vi "Save_Destinations.vi"(8 "error in (no error)":errorcluster, 11 "Installer in":refnum<class "Installer.lvclass">) -> (0 "error out":errorcluster, 3 "Installer out":refnum<class "Installer.lvclass">)   [LabVIEW 2020, in "Installer.lvclass"]
uses:
  <vilib>/AppBuilder/IB_Classes/Installer/Installer.lvclass
  <vilib>/AppBuilder/IB_Classes/Installer/Installer.lvclass/Installer.ctl
  <vilib>/AppBuilder/IB_Classes/Destination/IB_Destination.lvclass
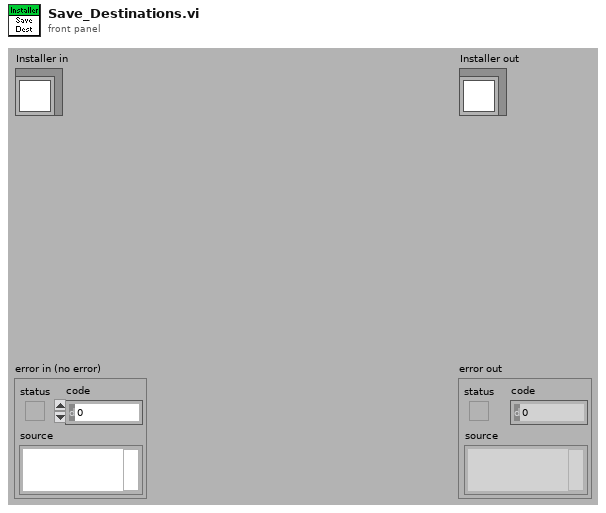
[diagram p1: front panel]
types:
  T1 = typedef "ItemRef.ctl" = u64
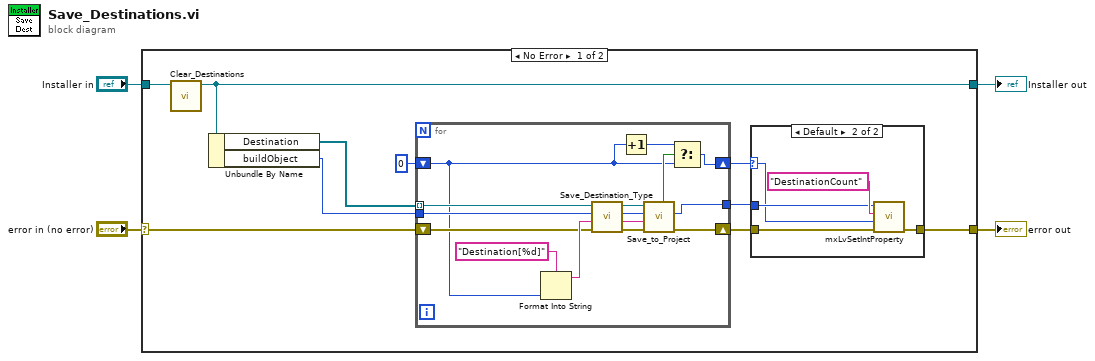
[diagram p0: block diagram]
diagram:
  n1 = case shown="No Error" "error in (no error)" {
    selector: "error in (no error)" -> [w7 w37]
    tunnel: [w6 w37] -> w3
    tunnel: [w12 w36] -> w1
    tunnel: "Installer in" -> [w13 w36]
    frame No Error {
      n2 = call <vilib>:"Clear_Destinations.vi"("Installer in"=w13) -> ("Installer out"=w12:refnum<class "Installer.lvclass">)  [unwired: 9 in, 1 out]
      n3 = Unbundle By Name(w12) -> ("Destination"=w14:refnum<class "IB_Destination.lvclass">[], "buildObject"=w11:T1)
      n4 = for {
        tunnel: w14 -> [w35] mode=indexing
        tunnel: w11 -> [w30]
        shift-right: [w27] -> w9
        shift-left: 0 -> [w21]
        shift-right: [w24] -> w8
        shift-left: w7 -> [w26]
        tunnel: [w23] -> w5
        n5 = Format Into String(format string="Destination[%d]", w21) -> (resulting string=w32:string)  [unwired: 2 in, 1 out]
        n6 = call-dynamic "Save_Destination_Type.vi"("error in (no error)"=w26, "index"=w32, "buildObject"=w30, "IB_Destination in"=w35) -> ("error out"=w25:errorcluster, "index out"=w31:string, "buildObject out"=w29:T1, "IB_Destination out"=w34:refnum<class "IB_Destination.lvclass">)  [unwired: 4 in]
        n7 = Increment(x=w21) -> (x+1=w28:i32)
        n8 = call-dynamic "Save_to_Project.vi"("error in (no error)"=w25, "index"=w31, "buildObject"=w29, "IB_Destination in"=w34) -> ("error out"=w24:errorcluster, "buildObject out"=w23:T1, "saved?"=w22:bool)  [unwired: 3 in, 2 out]
        n9 = Select(t=w28, s=w22, f=w21) -> (s? t:f=w27:i32)
      }
      n10 = case shown="Default" w9 {
        selector: w9 -> [_ w16]
        tunnel: w5 -> [_ w19]
        tunnel: w8 -> [w15 w18]
        tunnel: [w15 w17] -> w6
        frame 0 {
        }
        frame Default {
          n11 = call <resource>:"mxLvSetIntProperty.vi"("error in"=w18, "Value (0)"=w16, "Tag"="DestinationCount", "Item"=w19) -> ("error out"=w17:errorcluster)  [unwired: 1 in, 6 out]
        }
      }
    }
    frame Error {
    }
  }
  "error out" <- w3
  "Installer out" <- w1
